vi "ConfigDIO.vi"(0 "Pump_1AI_1DO_2DI in":refnum<class "Engine_1DO_2DI.lvclass">, 5 "DO":T2 items=["DO 0 [KP1] [M12]", "DO 1 [ON KP2] [M21]", "DO 2 [ON KP3] [M24]", "DO 3 [WATER Y18.1 [DO3]]", "DO 4 [WATER Y18.2 [DO4]]", "DO 5 [KP6 Y29.1 33.7]", "DO 6 [KP7 Y29.2 33.8]", "DO 7 [KP8 Y29.3 33.9]", "DO 8 [KP9 Y29.4  33.12]", "DO 9 [KP10 Y29.5 33.1]", "DO 10 [KP11 Y29.6 33.2]", "DO 11 [KP12 Y29.7  33.13]", "DO 12 [KP13 Y29.8  33.11]", "DO 13 [KP14 Y29.9 33.10]", "DO 14 [KP15 Y29.10  33.6]", "DO 15 [KP16 Y29.11  33.5]", "DO 16 [KP17 Y29.12  33.4]", "DO 17 [KP18 Y29.13 33.3]", "DO 18 [AIR KP19]", "DO 19 [STEP DRIVE EN KP20]", "DO 20 [KP21 Y44.1 OPEN]", "DO 21 [ KP22 Y44.1 CLOSE]", "DO 22 [ KP23 Y44.2 OPEN]", "DO 23", "DO 24 [STEP DRIVE 1]", "DO 25 [STEP DRIVE 2]"], 7 "DI A":T1 items=["DI 0 [QF1]", "DI 1 [QF2]", "DI 2 [QF3]", "DI 3 [QF4]", "DI 4 [QF5]", "DI 5 [QF6]", "DI 6 [QF7]", "DI 7 [QF8]", "DI 8 [QF9]", "DI 9 [PHASE CONTROL RELAY CONTACTOR [KV1]]", "DI 10 [G1]", "DI 11 [G2]", "DI 12 [RESET BTN [SB1]]", "DI 13 [START BTN [SB2]]", "DI 14 [STOP BTN [SB3]]", "DI 15 [ES BTN [SB4]]", "DI 16 [MANUAL/AUTO MODE SA1]", "DI 17 [[S1]]", "DI 18 [[S2]]", "DI 19 [[S3]]", "DI 20 [[S4]]", "DI 21 [44.1 OPEN]", "DI 22 [44.1 CLOSE]", "DI 23 [CONTACTOR [MK1]] M12", "DI 24 [AUTOMATIC [QF11]] M12", "DI 25 [CONTACTOR [MK2]] M21", "DI 26 [AUTOMATIC [QF12]] M21", "DI 27 [CONTACTOR [MK3]] M24", "DI 28 [AUTOMATIC [QF13]] M24", "DI 29 [44.2 OPEN]", "DI 30 [44.2 CLOSE]"], 9 "DI C":T1 items=["DI 0 [QF1]", "DI 1 [QF2]", "DI 2 [QF3]", "DI 3 [QF4]", "DI 4 [QF5]", "DI 5 [QF6]", "DI 6 [QF7]", "DI 7 [QF8]", "DI 8 [QF9]", "DI 9 [PHASE CONTROL RELAY CONTACTOR [KV1]]", "DI 10 [G1]", "DI 11 [G2]", "DI 12 [RESET BTN [SB1]]", "DI 13 [START BTN [SB2]]", "DI 14 [STOP BTN [SB3]]", "DI 15 [ES BTN [SB4]]", "DI 16 [MANUAL/AUTO MODE SA1]", "DI 17 [[S1]]", "DI 18 [[S2]]", "DI 19 [[S3]]", "DI 20 [[S4]]", "DI 21 [44.1 OPEN]", "DI 22 [44.1 CLOSE]", "DI 23 [CONTACTOR [MK1]] M12", "DI 24 [AUTOMATIC [QF11]] M12", "DI 25 [CONTACTOR [MK2]] M21", "DI 26 [AUTOMATIC [QF12]] M21", "DI 27 [CONTACTOR [MK3]] M24", "DI 28 [AUTOMATIC [QF13]] M24", "DI 29 [44.2 OPEN]", "DI 30 [44.2 CLOSE]"]) -> (4 "Pump_1AI_1DO_2DI out":refnum<class "Engine_1DO_2DI.lvclass">)   [LabVIEW 2019]
uses:
  Engine_1DO_2DI.lvclass
  C:/Users/H4001/Documents/GitHub/H4000/src/Device_class/Device.lvclass
  C:/Users/H4001/Documents/GitHub/H4000/src/Proccess_class/Proccess.lvclass
  FPGA/TypeDef/DO index.ctl
  FPGA/TypeDef/DI index.ctl
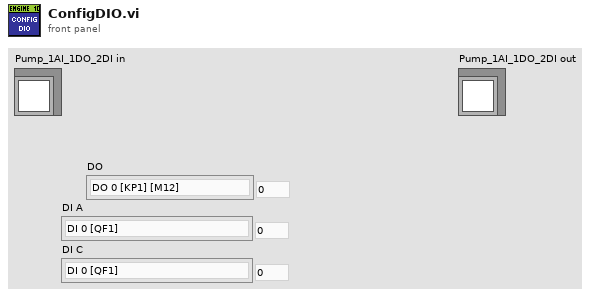
[diagram p1: front panel]
types:
  T1 = typedef "DI index.ctl" = u8
  T2 = typedef "DO index.ctl" = u8
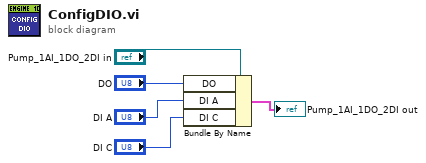
[diagram p0: block diagram]
diagram:
  n1 = Bundle By Name(cluster="Pump_1AI_1DO_2DI in", "DO"="DO", "DI A"="DI A", "DI C"="DI C") -> (→"Pump_1AI_1DO_2DI out":cluster{})
